vi "Do Get Open VIs.vi"(8 "error in (no error)":errorcluster, 10 "Get open VIs Argument":T3, 11 "Data Cluster 2":T1) -> (0 "error out":errorcluster, 3 "Data Cluster":T1)   [LabVIEW 2025, in "Scripting Server.lvlib"]
uses:
  Scripting Server.lvlib
  Get open VIs Argument--cluster.ctl
  Get open VIs (Reply Payload)--cluster.ctl
  Module Data--cluster.ctl
  Config Data.ctl
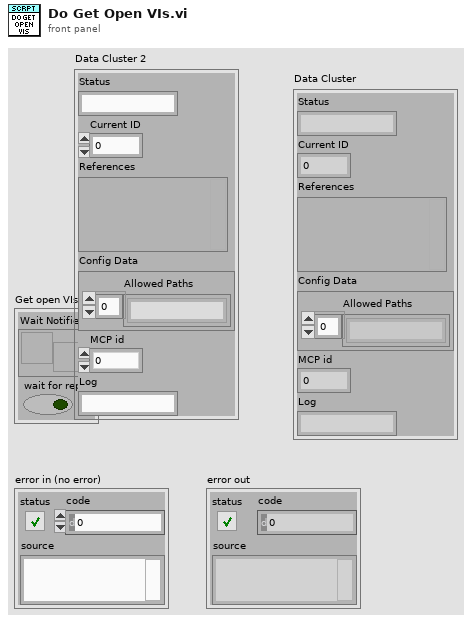
[diagram p1: front panel]
types:
  T1 = typedef "Scripting Server.lvlib/Module Data--cluster.ctl" = cluster{"Status":string, "Current ID":i32, "References":variant, "Config Data":T2, "MCP id":i32, "Log":string}
  T2 = typedef "Scripting Server.lvlib/Config Data.ctl" = cluster{"Allowed Paths":string[]}
  T3 = typedef "Scripting Server.lvlib/Get open VIs Argument--cluster.ctl" = cluster{"Wait Notifier":refnum<notifier>, "wait for reply":bool}
  T4 = typedef "Scripting Server.lvlib/Get open VIs (Reply Payload)--cluster.ctl" = cluster{"IDs":i32[], "Names":string[], "error":errorcluster}
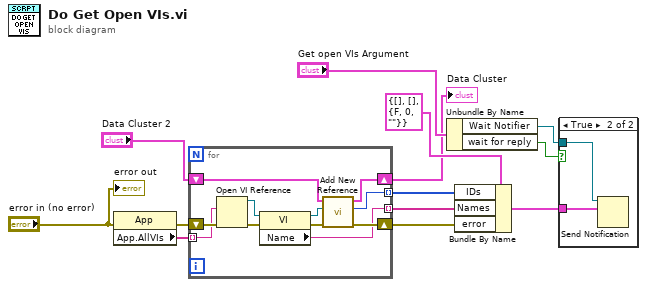
[diagram p0: block diagram]
diagram:
  n1 = property class="App"(error in="error in (no error)") -> (error out=w8:errorcluster, "App.AllVIs"=w5:string[])  [unwired: 1 in, 1 out]
  n2 = for {
    shift-right: [w23] -> w1
    shift-left: w8 -> [w24]
    shift-right: [w21] -> w6
    shift-left: "Data Cluster 2" -> [w22]
    tunnel: w5 -> [w19] mode=indexing
    tunnel: [w18] -> w4 mode=indexing
    tunnel: [w14] -> w3 mode=indexing
    n3 = Open VI Reference(vi path=w19, error in (no error)=w24) -> (vi reference=w16:refnum<vi>, error out=w20:errorcluster)  [unwired: 4 in]
    n4 = property class="VI"(reference=w16, error in=w20) -> (reference out=w15:refnum<vi>, error out=w17:errorcluster, "Name"=w14:string)
    n5 = call "Add New Reference.vi"("error in (no error)"=w17, "Variant"=w15, "Data Cluster in"=w22) -> ("error out"=w23:errorcluster, "new reference"=w18:i32, "Data Cluster out 2"=w21:T1)  [unwired: 6 in]
  }
  "Data Cluster" <- w6
  n6 = Unbundle By Name("Get open VIs Argument") -> ("Wait Notifier"=w10:refnum<notifier>, "wait for reply"=w11:bool)
  n7 = Bundle By Name(cluster=T4 {"IDs"=[], "Names"=[], "error"={"status"=FALSE, "code"=0, "source"=""}} ("Get open VIs (Reply Payload)"), "IDs"=w4, "Names"=w3, "error"=w1) -> (w12:T4)
  n8 = case "DQMH_FIRE_NOTIFIER" shown="True" w11 {
    tunnel: w10 -> [_ w26]
    tunnel: w12 -> [_ w25]
    frame False {
    }
    frame True {
      n9 = Send Notification(notification=w25, notifier=w26) -> ()  [unwired: 1 in, 2 out]
    }
  }
  "error out" <- "error in (no error)"
